vi "out.vi"(1 "Async ?":bool, 5 "IN VARIANT":variant, 7 "Ip":string, 9 "Name in":string, 11 "error in (no error)":errorcluster) -> (10 "Operation Ok":bool, 15 "error out":errorcluster)   [LabVIEW 2015]
doc: "Write the tuple (variant) \"name\" in the tuple space."
uses:
  C:/Users/Giuseppe/Downloads/LabLinda_ pakage/index_datatype.ctl
  C:/Users/Giuseppe/Downloads/LabLinda_ pakage/index_cluster.ctl
  LI_states.ctl
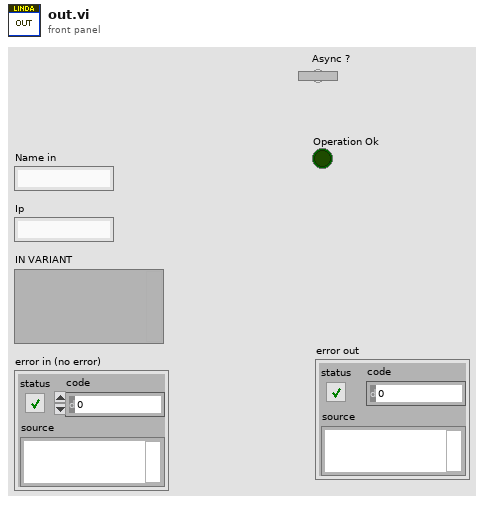
[diagram p1: front panel]
types:
  T1 = typedef "LI_states.ctl" = enum16{"Out", "In", "Rd", "Inp", "Rdp", "Init", "Cleanup", "RdAll"}
  T2 = typedef "index_datatype.ctl" = T3[]
  T3 = typedef "index_cluster.ctl" = cluster{"Addr":i32[], "out react vi reference":refnum<vi>, "in react vi reference":refnum<vi>, "rd react vi reference":refnum<vi>, "Read_write_var":refnum<vi>}
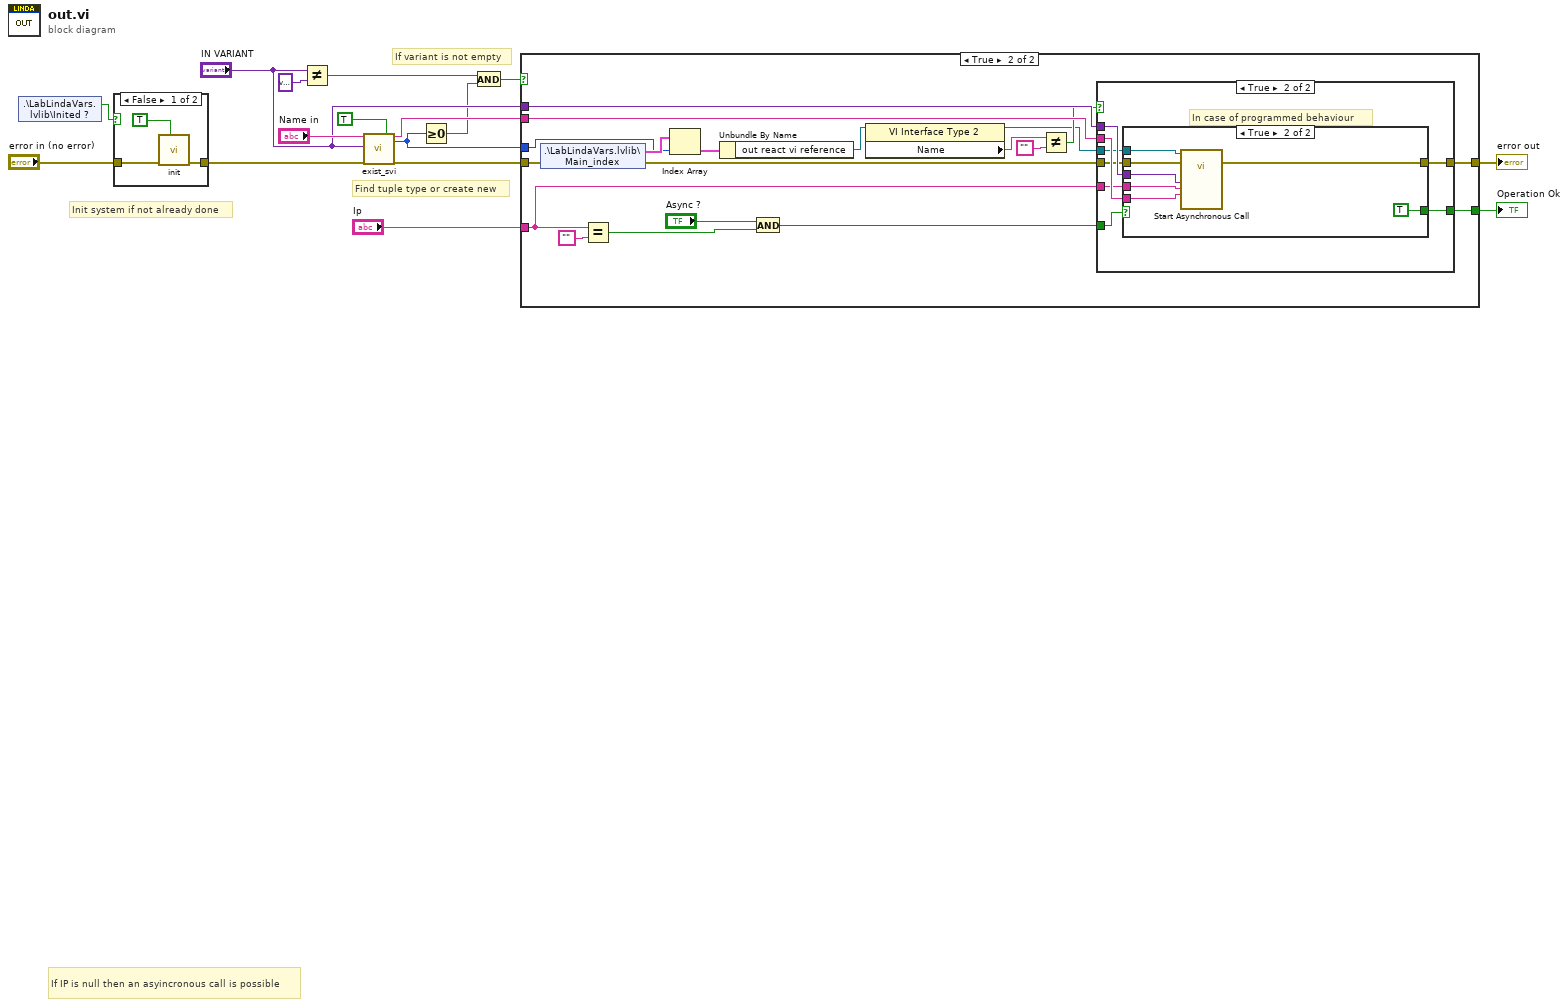
[diagram p0: block diagram]
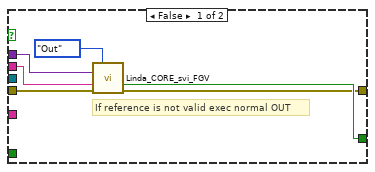
[diagram p3: hidden frame]
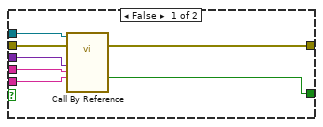
[diagram p4: hidden frame]
diagram:
  # "If variant is not empty"
  # "If IP is null then an asyincronous call is possible"
  # "Init system if not already done"
  # "Find tuple type or create new"
  n1 = shared-variable ".\\LabLindaVars.lvlib\\Inited ?"() -> (w13:bool)  [unwired: 1 in, 1 out]
  n2 = case shown="False" w13 {
    tunnel: [w19 w20] -> w7
    tunnel: "error in (no error)" -> [w18 w20]
    frame False {
      n3 = call "init.vi"("Cleaneup"=TRUE, "error in (no error)"=w18) -> ("error out"=w19:errorcluster)  [unwired: 9 in]
    }
    frame True {
    }
  }
  n4 = Not Equal?(x="IN VARIANT", y=variant ("IN VARIANT")) -> (x != y?=w2:bool)
  n5 = call "exist_svi.vi"("Name"="Name in", "IN VARIANT"="IN VARIANT", "error in (no error)"=w7, "Create ?"=TRUE) -> ("Name"=w14:string, "index of element"=w6:i32, "error out"=w8:errorcluster)  [unwired: 12 in, 1 out]
  n6 = Greater Or Equal To 0?(x=w6) -> (x >= 0?=w3:bool)
  n7 = And(x=w2, y=w3) -> (x .and. y?=w1:bool)
  n8 = case shown="True" w1 {
    tunnel: w14 -> [_ w38]
    tunnel: "IN VARIANT" -> [_ w37]
    tunnel: [_ w31] -> w11
    tunnel: [w21 w30] -> w10
    tunnel: "Ip" -> [_ w26]
    tunnel: w8 -> [w21 w23]
    tunnel: w6 -> [_ w22]
    frame False {
    }
    frame True {
      n9 = shared-variable ".\\LabLindaVars.lvlib\\Main_index"(error in=w23) -> (w39:T2, error out=w36:errorcluster)
      n10 = Equal?(x=w26, y="") -> (x = y?=w25:bool)
      n11 = Index Array(array=w39, index=w22) -> (element=w40:T3)
      n12 = Unbundle By Name(w40) -> ("out react vi reference"=w35:refnum<vi>)
      n13 = And(x="Async ?", y=w25) -> (x .and. y?=w24:bool)
      n14 = property class="VI Interface Type 2"(reference=w35) -> (reference out=w29:refnum<vi>, "Name"=w34:string)  [unwired: 1 in, 1 out]
      n15 = Not Equal?(x=w34, y="") -> (x != y?=w32:bool)
      n16 = case shown="True" w32 {
        tunnel: w38 -> [w44 w54]
        tunnel: w37 -> [w45 w53]
        tunnel: w36 -> [w41 w52]
        tunnel: w29 -> [_ w51]
        tunnel: [w43 w50] -> w31
        tunnel: [w42 w49] -> w30
        tunnel: w26 -> [_ w48]
        tunnel: w24 -> [_ w47]
        frame False {
          # "If reference is not valid exec normal OUT"
          n17 = call "Linda_CORE_svi_FGV.vi"("OP"=LI_states."Out", "IN VARIANT"=w45, "Name in"=w44, "error in (no error)"=w41) -> ("Valid Op"=w43:bool, "error out"=w42:errorcluster)  [unwired: 7 in, 3 out]
        }
        frame True {
          # "In case of programmed behaviour"
          n18 = case shown="True" w47 {
            tunnel: w51 -> [w61 w68]
            tunnel: w53 -> [w58 w67]
            tunnel: w54 -> [w60 w65]
            tunnel: w48 -> [w59 w66]
            tunnel: [w55 TRUE ("Operation Ok")] -> w50
            tunnel: w52 -> [w57 w62]
            tunnel: [w56 w63] -> w49
            frame False {
              n19 = call-by-ref "?"(reference=w61, error in=w57, "IN VARIANT"=w58, "Ip"=w59, "Name in"=w60) -> (error out=w56:errorcluster, "Operation Ok"=w55:bool)  [unwired: 11 in, 2 out]
            }
            frame True {
              n20 = call-by-ref "Start Asynchronous Call"(reference=w68, error in=w62, "IN VARIANT"=w67, "Ip"=w66, "Name in"=w65) -> (error out=w63:errorcluster)  [unwired: 11 in, 3 out]
            }
          }
        }
      }
    }
  }
  "Operation Ok" <- w11
  "error out" <- w10
